vi "Gyro.vi"(7 "Action":T4, 8 "error in":errorcluster, 9 "Gain (VoltsPerDegree/Second)":dbl=0.007, 11 "GyroDevRef":T1={"DevStatus"={"status"=FALSE, "code"=0, "source"=""}, "Analog Module"=enum."Analog Module 2", "Analog Channel"=enum."AI 1", "Offset"=0.0, "Gain (VoltsPerDegree/Second)"=0.0}) -> (0 "error out":errorcluster, 3 "Angle":dbl(knob) scale=0.0..360.0)   [LabVIEW 2013]
doc: "Wrapper for the gyro. It has the following actions:\n-Init: initialize a gyro reference with the given analog module, analog channel, and gain.\n-ReadAngle: returns the gyro angle mod 360."
uses:
  Read Angle Mode.ctl
  <vilib>/Rock Robotics/WPI/Gyro/WPI_GyroDevRef.ctl
  <vilib>/Rock Robotics/SystemInterfaces/Typedef/FPGA_TypedefAnalogModule.ctl
  <vilib>/Rock Robotics/SystemInterfaces/AI/FPGA_AIChannel.ctl
panel:
  # "This will display the current gyro angle."
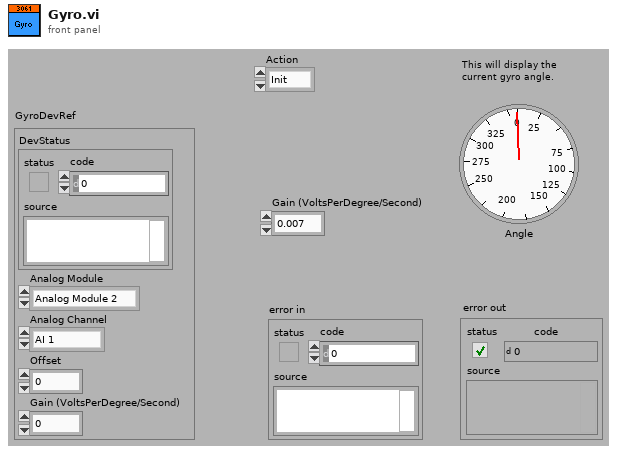
[diagram p1: front panel]
types:
  T1 = typedef "WPI_GyroDevRef.ctl" = cluster{"DevStatus":errorcluster, "Analog Module":T2, "Analog Channel":T3, "Offset":dbl, "Gain (VoltsPerDegree/Second)":dbl}
  T2 = typedef "FPGA_TypedefAnalogModule.ctl" = enum16{"Analog Module 1", "Analog Module 2"}
  T3 = typedef "FPGA_AIChannel.ctl" = enum8{"AI 1", "AI 2", "AI 3", "AI 4", "AI 5", "AI 6", "AI 7", "AI 8", "Invalid"}
  T4 = typedef "Read Angle Mode.ctl" = enum16{"Init", "ReadAngle", "Disable"}
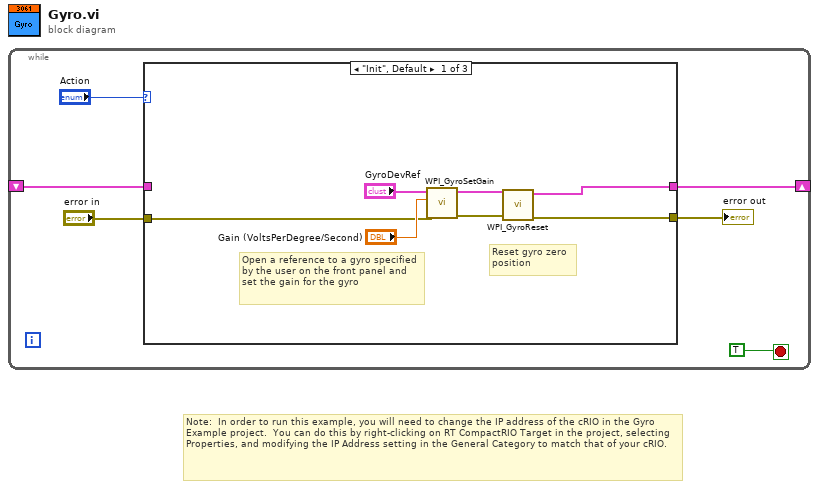
[diagram p0: block diagram]
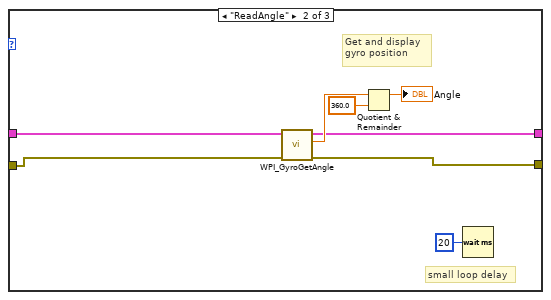
[diagram p2: hidden frame]
diagram:
  # "Note:  In order to run this example, you will need to change the IP address of the cRIO in the Gyro Example project.  You can do this by right-clicking on RT CompactRIO Target in the project, selecting Properties, and modifying the IP Address setting in the General Category to match that of your cRIO."
  n1 = while {
    shift-right: [w5] -> _
    shift-left: _ -> [w6]
    stop <- TRUE stop-if-true
    n2 = case shown="\"Init\", Default" "Action" {
      tunnel: w6 -> [_ w15 w23]
      tunnel: [w11 w20 w23] -> w5
      tunnel: [w9 w16 w22] -> w2
      tunnel: "error in" -> [w8 w14 w22]
      frame "Init", Default {
        # "Reset gyro zero \nposition"
        # "Open a reference to a gyro specified by the user on the front panel and set the gain for the gyro"
        n3 = call <vilib>:"WPI_GyroSetGain.vi"("error in (no error)"=w8, "Gain (VoltsPerDegree/Second)"="Gain (VoltsPerDegree/Second)", "GyroDevRef"="GyroDevRef") -> ("error out"=w10:errorcluster, "GyroDevRef"=w12:T1)  [unwired: 7 out]
        n4 = call <vilib>:"WPI_GyroReset.vi"("error in (no error)"=w10, "GyroDevRef"=w12) -> ("error out"=w9:errorcluster, "GyroDevRef"=w11:T1)  [unwired: 8 out]
      }
      frame "ReadAngle" {
        # "small loop delay"
        # "Get and display\ngyro position"
        n5 = call <vilib>:"WPI_GyroGetAngle.vi"("error in (no error)"=w14, "GyroDevRef"=w15) -> ("error out"=w16:errorcluster, "Angle"=w21:dbl, "GyroDevRef"=w20:T1)  [unwired: 7 out]
        n6 = Quotient & Remainder(x=w21, y=360.0) -> (x-y*floor(x/y)=→"Angle":dbl)  [unwired: 1 out]
        n7 = Wait (ms)(milliseconds to wait=u32 20) -> ()  [unwired: 1 out]
      }
      frame "Disable" {
        # "Close the reference\nto the gyro"
      }
    }
    "error out" <- w2
  }
